vi "TRStimestampCheck.vi"(10 "element":u32 format="%032b") -> (2 "TRSTimestamp?":bool)   [LabVIEW 2014]
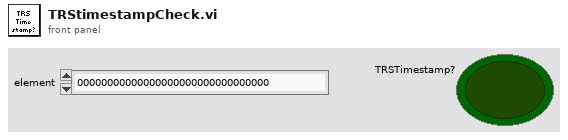
[diagram p1: front panel]
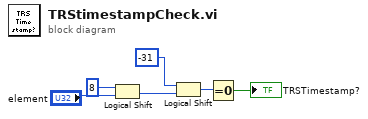
[diagram p0: block diagram]
diagram:
  n1 = Logical Shift(y=i16 8, x="element") -> (x << y=w3:u32)
  n2 = Logical Shift(y=i16 -31, x=w3) -> (x << y=w2:u32)
  n3 = Equal To 0?(x=w2) -> (x = 0?=→"TRSTimestamp?":bool)
